vi "CheesyDrive.vi"(6 "Quickturn":bool, 8 "QuickTurn Sensitivty":dbl=0.7, 9 "Sensitivty":dbl=0.5, 10 "Wheel":dbl(slide) scale=-1.0..1.0, 11 "Throttle":dbl(slide) scale=-1.0..1.0) -> (2 "Right PWM":dbl, 3 "Left PWM":dbl)   [LabVIEW 2019]
panel:
  out "Waveform Chart 2":cluster{"left":dbl, "right":dbl}(graph)
  in  "alpha":dbl=0.1
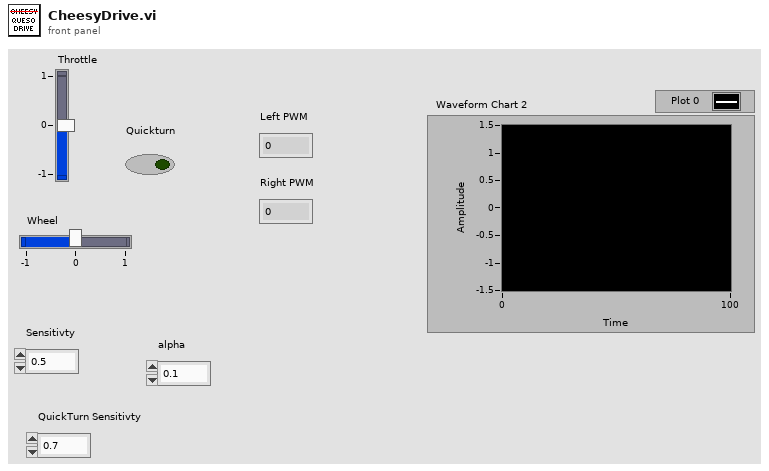
[diagram p1: front panel]
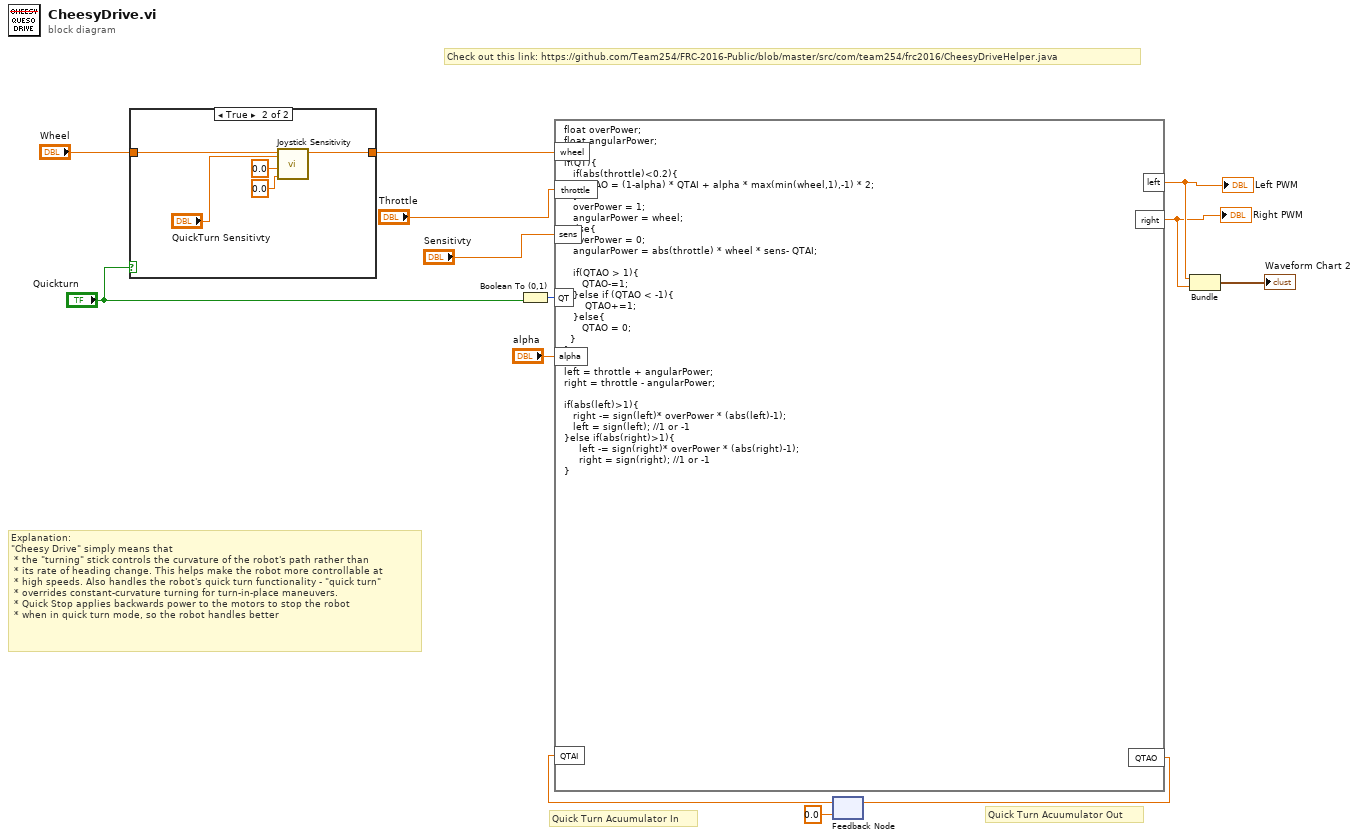
[diagram p0: block diagram]
diagram:
  # "Explanation:\n\"Cheesy Drive\" simply means that\n * the \"turning\" stick controls the curvature of the robot's path rather than\n * its rate of heading change. This helps make the robot more controllable at\n * high speeds. Also handles the robot's quick turn functionality - \"quick turn\"\n * overrides constant-curvature turning for turn-in-place maneuvers.\n * Quick Stop applies backwards power to the motors to stop the robot\n * when in quick turn mode, so the robot handles better"
  # "Quick Turn Acuumulator Out"
  # "Quick Turn Acuumulator In"
  # "Check out this link: https://github.com/Team254/FRC-2016-Public/blob/master/src/com/team254/frc2016/CheesyDriveHelper.java"
  n1 = case shown="True" "Quickturn" {
    tunnel: "Wheel" -> [w14 w19]
    tunnel: [w14 w18] -> w1
    frame False {
    }
    frame True {
      n2 = call "Joystick Sensitivity.vi"("joystick deadband"=0.0, "motor deadband (0.15)"=0.0, "sensitivity (0.5)"="QuickTurn Sensitivty", "x"=w19) -> ("y"=w18:dbl)  [unwired: 6 in, 1 out]
    }
  }
  n3 = Boolean To (0,1)(Boolean="Quickturn") -> (0, 1=w11:i16)
  n4 = feedback #1(0.0 ("QTAccumulatorO")) -> (w9:dbl)
  n5 = formula code="float overPower;\nfloat angularPower;\n\nif(QT){\n   if(abs(throttle)<0.2){\n      QTAO = (1-alpha) * QTAI + alpha * max(min(wheel,1),-1) * 2;\n   }\n   overPower = 1;\n   angularPower = wheel;\n}else{\n   overPower = 0;\n   angularPower = abs(throttle) * wheel * sens- QTAI;\n\n   if(QTAO > 1){\n      QTAO-=1;\n   }else if (QTAO < -1){\n       QTAO+=1;\n   }else{\n      QTAO = 0;\n  }\n}\n\nleft = throttle + angularPower;\nright = throttle - angularPower;\n\nif(abs(left)>1){\n   right -= sign(left)* overPower * (abs(left)-1);\n   left = sign(left); //1 or -1\n}else if(abs(right)>1){\n     left -= sign(right)* overPower * (abs(right)-1);\n     right = sign(right); //1 or -1 \n}"("wheel"=w1, "throttle"="Throttle", "sens"="Sensitivty", "QT"=w11, "alpha"="alpha", "QTAI"=w9) -> ("left"=w6:dbl, "right"=w5:dbl, "QTAO"=w12:dbl)
  "Left PWM" <- w6
  "Right PWM" <- w5
  n6 = feedback-in #1(w12) -> ()
  n7 = Bundle("left"=w6, "right"=w5) -> (→"Waveform Chart 2":cluster{"left":dbl, "right":dbl})  [unwired: 1 in]
